vi "Get Default Reference.vi"(4 "Grid Size":cluster{"Max X":u32, "Max Y":u32}={"Max X"=3, "Max Y"=3}, 6 "Grid Descriptor":cluster{"X Step":sgl, "Y Step":sgl, "Unit":T2}, 8 "error in (no error)":errorcluster, 9 "Reference Points":T3, 11 "Image In":T1) -> (0 "error out":errorcluster, 1 "Default Real Reference":cluster{"X":dbl, "Y":dbl}[](array[cluster]), 2 "Pixel Reference":cluster{"X":dbl, "Y":dbl}[](array[cluster]), 3 "Image Out":T1)   [LabVIEW 2015]
uses:
  <vilib>/vision/Calibration.llb/Calibration Reference Points.ctl
  <vilib>/vision/Image Controls.llb/IMAQ Image.ctl
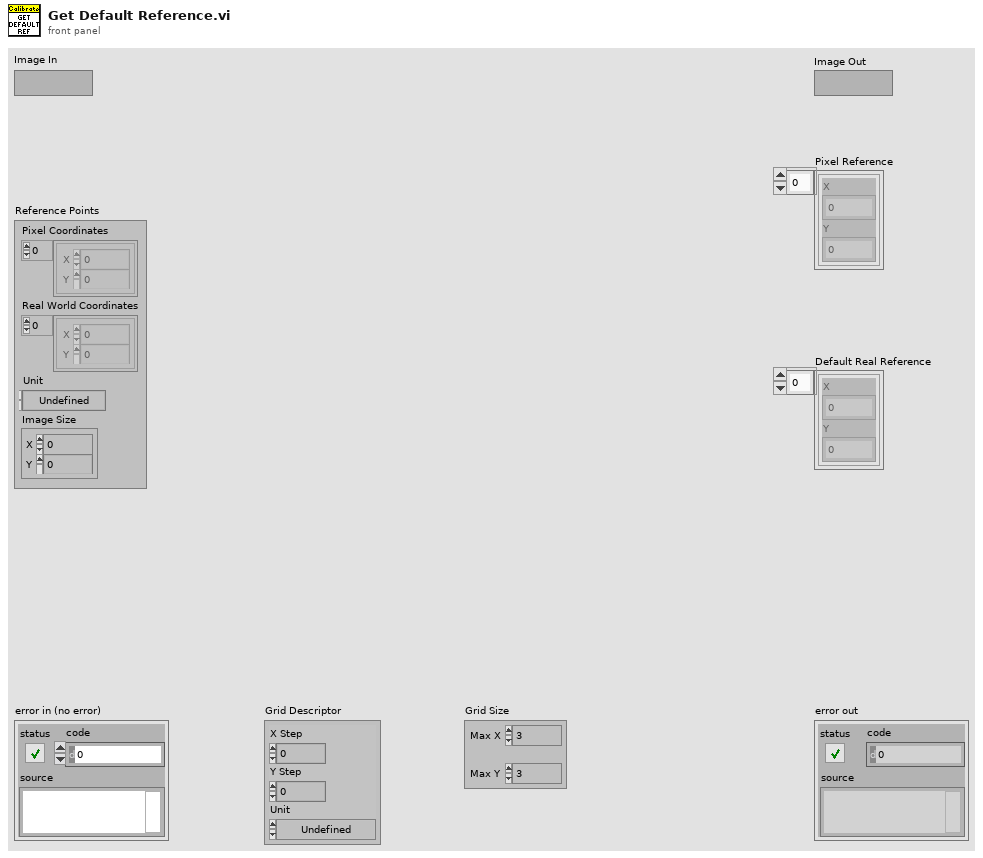
[diagram p1: front panel]
types:
  T1 = typedef "IMAQ Image.ctl" = refnum<image>
  T2 = typedef "Image Unit" = enum32{"Undefined", "Angström", "Micrometer", "Millimeter", "Centimeter", "Meter", "Kilometer", "Microinch", "Inch", "Feet", "Nautical miles", "Standard miles", "Steps"}
  T3 = typedef "Calibration Reference Points.ctl" = cluster{"Pixel Coordinates":cluster{"X":dbl, "Y":dbl}[], "Real World Coordinates":cluster{"X":dbl, "Y":dbl}[], "Unit":T2, "Image Size":cluster{"X":u32, "Y":u32}}
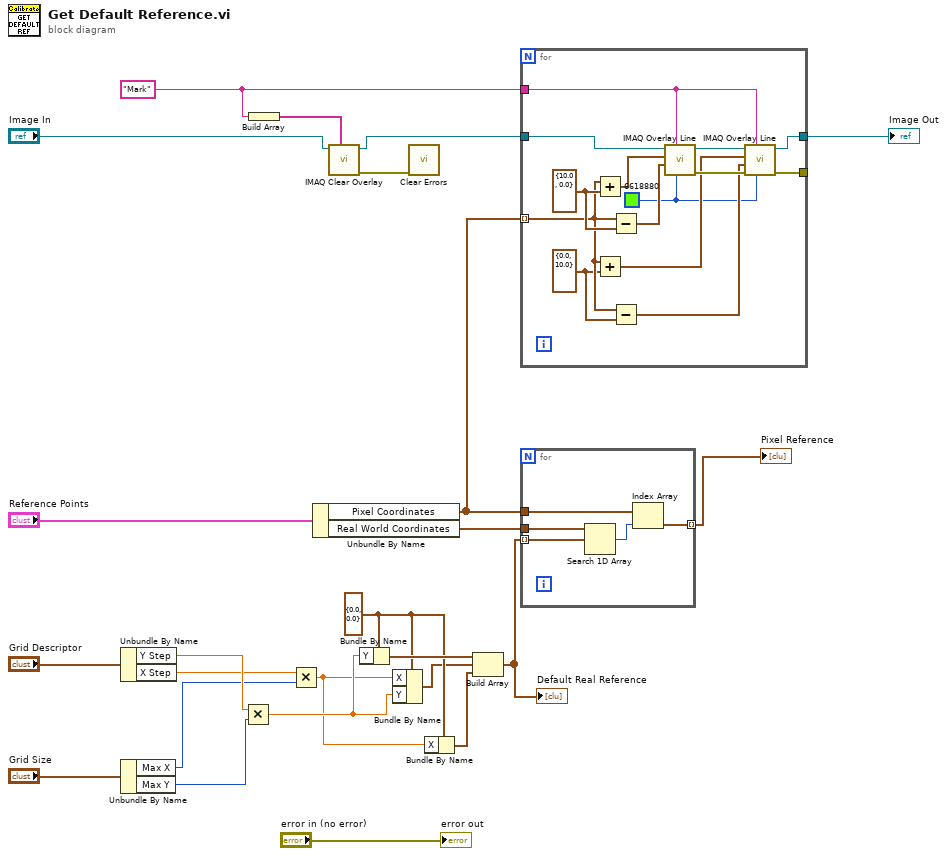
[diagram p0: block diagram]
diagram:
  w5 = "Mark" ("Group")
  w14 = cluster{"X":dbl, "Y":dbl} {"X"=0.0, "Y"=0.0} ("Reference Points")
  n1 = Unbundle By Name("Grid Descriptor") -> ("Y Step"=w16:sgl, "X Step"=w15:sgl)
  n2 = Unbundle By Name("Grid Size") -> ("Max X"=w1:u32, "Max Y"=w2:u32)
  n3 = Multiply(x=w16, y=w2) -> (x*y=w9:sgl)
  n4 = Build Array(w5) -> (w4:string[])
  n5 = Multiply(x=w15, y=w1) -> (x*y=w8:sgl)
  n6 = Unbundle By Name("Reference Points") -> ("Pixel Coordinates"=w11:cluster{"X":dbl, "Y":dbl}[], "Real World Coordinates"=w22:cluster{"X":dbl, "Y":dbl}[])
  n7 = call "IMAQ Clear Overlay"("Groups"=w4, "Image"="Image In") -> ("error out"=w3:errorcluster, "Image Out"=w7:T1)  [unwired: 8 in]
  n8 = Bundle By Name(cluster=w14, "Y"=w9) -> (w20:cluster{"X":dbl, "Y":dbl})
  n9 = Bundle By Name(cluster=w14, "X"=w8, "Y"=w9) -> (w12:cluster{"X":dbl, "Y":dbl})
  n10 = call <vilib>:"Clear Errors.vi"("error in (no error)"=w3) -> ()  [unwired: 5 in, 2 out]
  n11 = Bundle By Name(cluster=w14, "X"=w8) -> (w13:cluster{"X":dbl, "Y":dbl})
  n12 = Build Array(w20, w12, w13) -> (w19:cluster{"X":dbl, "Y":dbl}[])
  "Default Real Reference" <- w19
  n13 = for {
    tunnel: w11 -> [w32] mode=indexing
    tunnel: w7 -> [w38]
    tunnel: [w28] -> _
    tunnel: [w26] -> w10
    tunnel: w5 -> [w25]
    w27 = u32 6618880 ("Color")
    w31 = cluster{"X":dbl, "Y":dbl} {"X"=0.0, "Y"=10.0} ("y")
    w33 = cluster{"X":dbl, "Y":dbl} {"X"=10.0, "Y"=0.0} ("y")
    n14 = Add(x=w32, y=w33) -> (x+y=w34:cluster{"X":dbl, "Y":dbl})
    n15 = Add(x=w32, y=w31) -> (x+y=w29:cluster{"X":dbl, "Y":dbl})
    n16 = Subtract(x=w32, y=w33) -> (x-y=w35:cluster{"X":dbl, "Y":dbl})
    n17 = Subtract(x=w32, y=w31) -> (x-y=w30:cluster{"X":dbl, "Y":dbl})
    n18 = call "IMAQ Overlay Line"("Color"=w27, "Group"=w25, "End Point"=w35, "Start Point"=w34, "Image"=w38) -> ("error out"=w36:errorcluster, "Image Out"=w37:T1)  [unwired: 5 in]
    n19 = call "IMAQ Overlay Line"("Color"=w27, "Group"=w25, "error in (no error)"=w36, "End Point"=w30, "Start Point"=w29, "Image"=w37) -> ("error out"=w28:errorcluster, "Image Out"=w26:T1)  [unwired: 4 in]
  }
  "Image Out" <- w10
  n20 = for {
    tunnel: w22 -> [w43]
    tunnel: w19 -> [w42] mode=indexing
    tunnel: w11 -> [w40]
    tunnel: [w39] -> w18 mode=indexing
    n21 = Search 1D Array(1D array=w43, element=w42) -> (index of element=w41:i32)  [unwired: 1 in]
    n22 = Index Array(array=w40, index=w41) -> (element=w39:cluster{"X":dbl, "Y":dbl})
  }
  "Pixel Reference" <- w18
  "error out" <- "error in (no error)"
